vi "cameraHandler.vi"() -> ()   [LabVIEW 2011]
panel:
  in  "camerahandler":i32
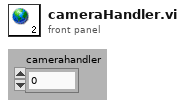
[diagram p1: front panel]
diagram:
